vi "e.gate Decode Summary File.vi"(8 "error in (no error)":errorcluster, 11 "e.gate Configuration In":T1) -> (0 "error out":errorcluster, 3 "e.gate Configuration Out":T1)   [LabVIEW 2016]
doc: "This VI reads all, for decoding relevant, data from #summary.sta ini file to the configuration cluster."
uses:
  e.gate Configuration.ctl
  e.gate Channel Data.ctl
  e.gate Data Type.ctl
  e.gate Protocol Type.ctl
  e.gate Module  Data.ctl
  e.gateHSP_DLLhandle.ctl
  <vilib>/Utility/config.llb/Read Key (String).vi
  <vilib>/Utility/config.llb/NI_LVConfig.lvlib
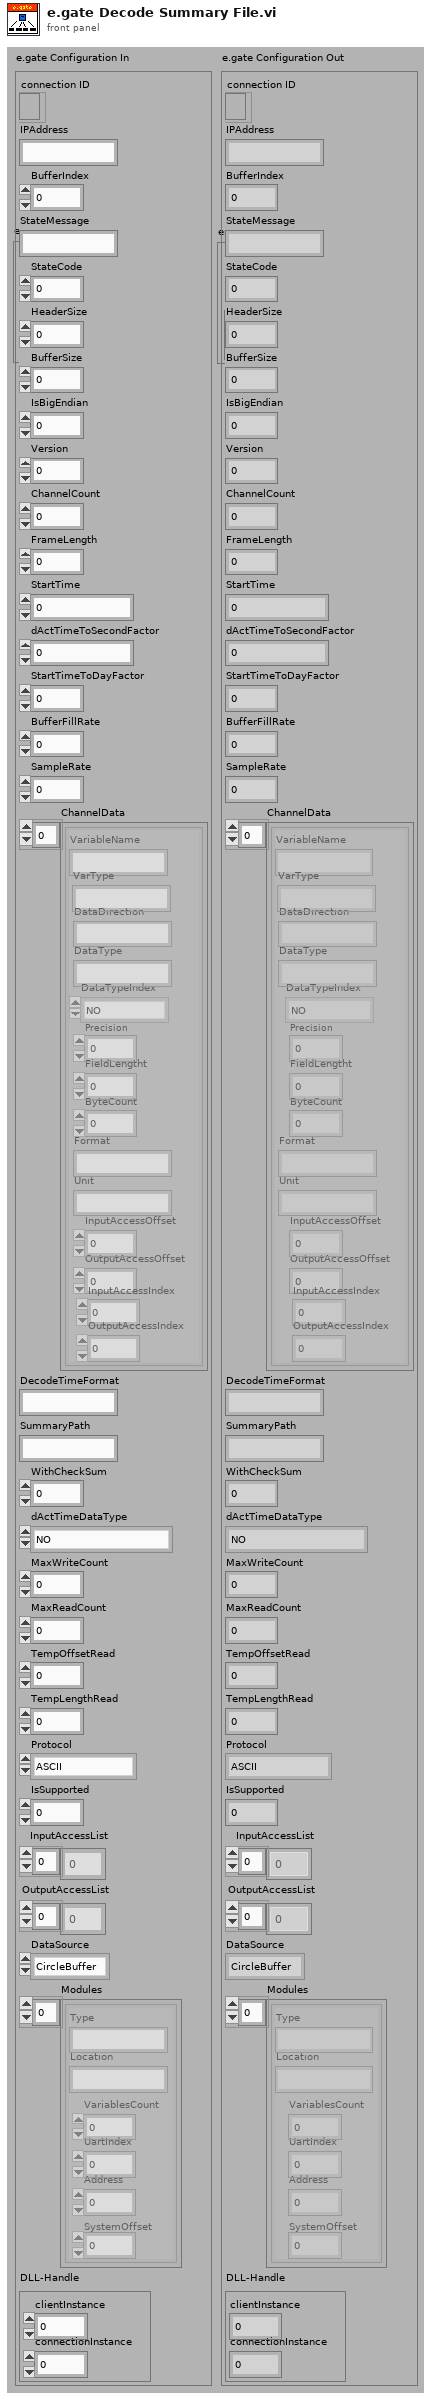
[diagram p1: front panel]
types:
  T1 = typedef "e.gate Configuration.ctl" = cluster{"connection ID":refnum<k5>, "IPAddress":string, "BufferIndex":i32, "StateMessage":string, "StateCode":i8, "HeaderSize":i32, "BufferSize":i32, "IsBigEndian":i32, "Version":i32, "ChannelCount":i32, "FrameLength":i32, "StartTime":dbl, "dActTimeToSecondFactor":dbl, "StartTimeToDayFactor":dbl, "BufferFillRate":dbl, "SampleRate":dbl, "ChannelData":T2[], "DecodeTimeFormat":string, "SummaryPath":string, "WithCheckSum":i32, "dActTimeDataType":T3, "MaxWriteCount":i32, "MaxReadCount":i32, "TempOffsetRead":i32, "TempLengthRead":i32, "Protocol":T4, "IsSupported":i32, "InputAccessList":i32[], "OutputAccessList":i32[], "DataSource":enum16{"CircleBuffer", "test.con Logger", "test.con Archive"}, "Modules":T5[], "DLL-Handle":T6}
  T2 = typedef "e.gate Channel Data.ctl" = cluster{"VariableName":string, "DataDirection":string, "DataType":string, "DataTypeIndex":T3, "Precision":i16, "FieldLengtht":i16, "ByteCount":i32, "Format":string, "Unit":string, "InputAccessOffset":i32, "OutputAccessOffset":i16, "InputAccessIndex":i16, "OutputAccessIndex":i16, "VarType":string}
  T3 = typedef "e.gate Data Type.ctl" = enum16{"NO", "BOOL", "SINT8", "USINT8", "SINT16", "USINT16", "SINT32", "USINT32", "FLOAT", "SET8", "SET16", "SET32", "DOUBLE", "SINT64", "USINT64", "SET64"}
  T4 = typedef "e.gate Protocol Type.ctl" = enum16{"ASCII", "HighspeedPort Online", "HighspeedPort Buffer", "eGateHighspeedPortDLL "}
  T5 = typedef "e.gate Module  Data.ctl" = cluster{"Type":string, "Location":string, "VariablesCount":i16, "UartIndex":i16, "Address":i16, "SystemOffset":i16}
  T6 = typedef "e.gateHSP_DLLhandle.ctl" = cluster{"clientInstance":i32, "connectionInstance":i32}
  T7 = typedef "NI_LVConfig.lvlib/Config Data RefNum.ctl" = refnum<k1>
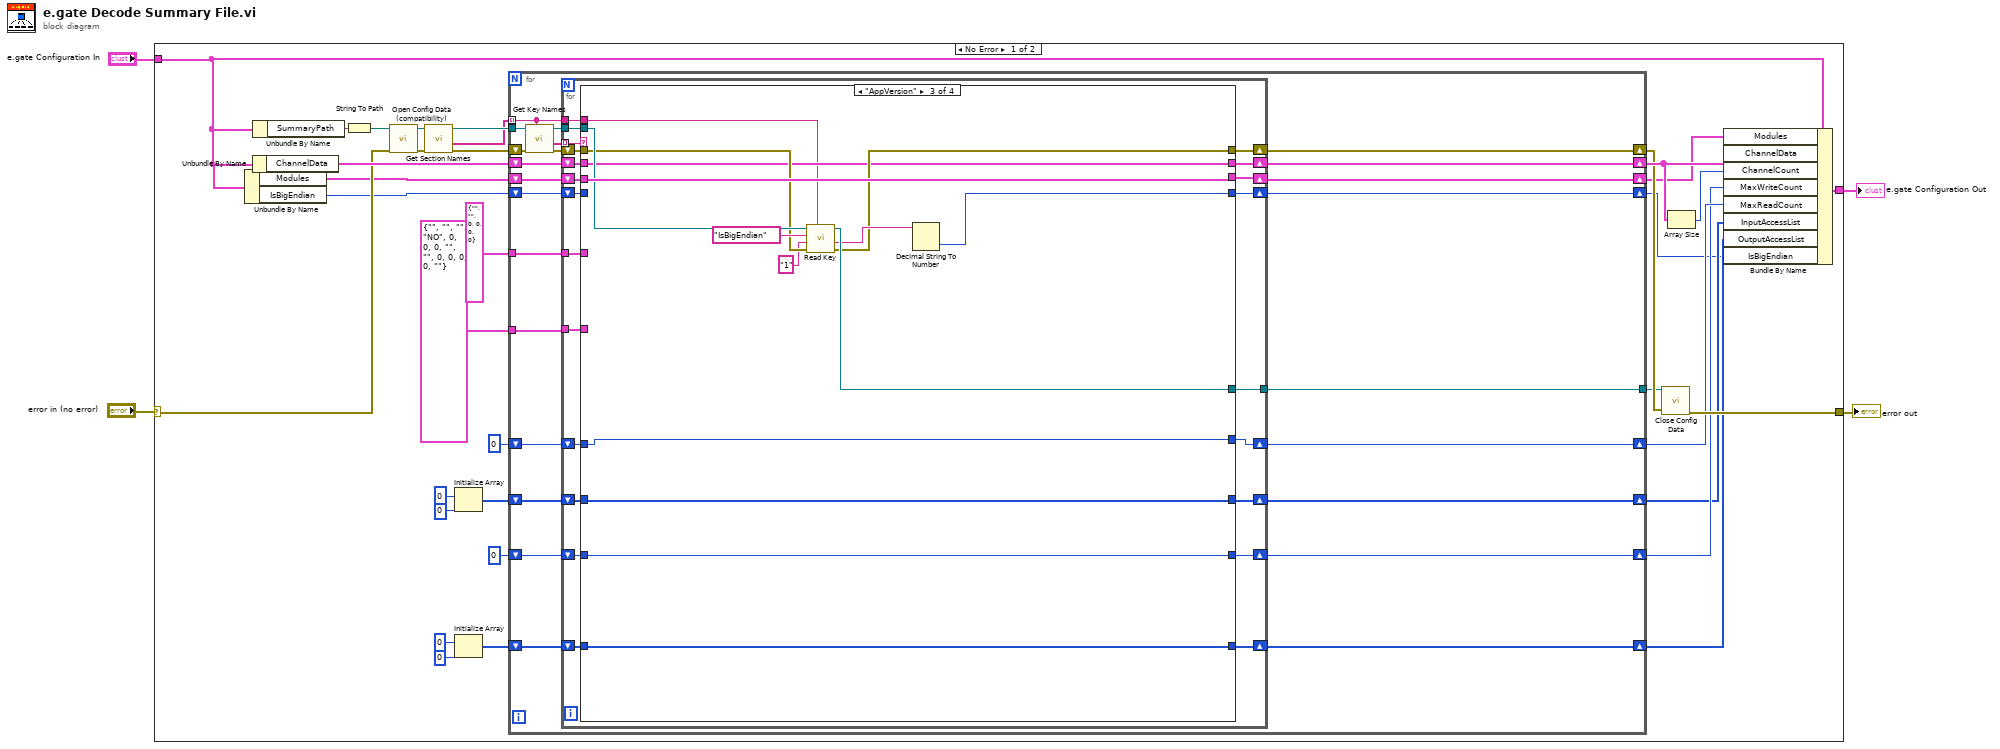
[diagram p0: block diagram]
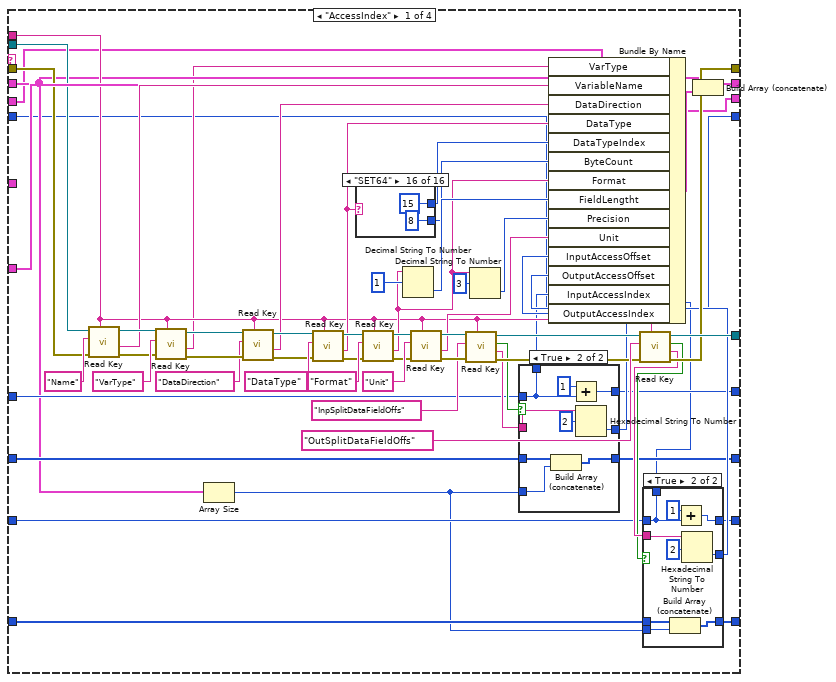
[diagram p2: hidden frame]
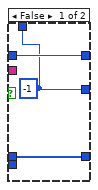
[diagram p3: hidden frame]
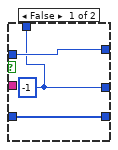
[diagram p4: hidden frame]
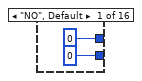
[diagram p5: hidden frame]
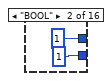
[diagram p6: hidden frame]
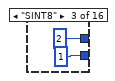
[diagram p7: hidden frame]
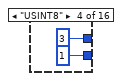
[diagram p8: hidden frame]
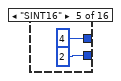
[diagram p9: hidden frame]
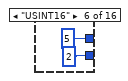
[diagram p10: hidden frame]
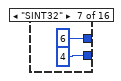
[diagram p11: hidden frame]
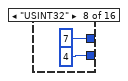
[diagram p12: hidden frame]
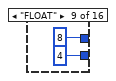
[diagram p13: hidden frame]
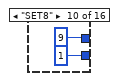
[diagram p14: hidden frame]
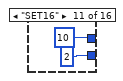
[diagram p15: hidden frame]
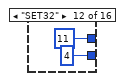
[diagram p16: hidden frame]
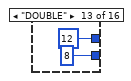
[diagram p17: hidden frame]
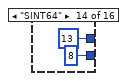
[diagram p18: hidden frame]
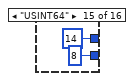
[diagram p19: hidden frame]
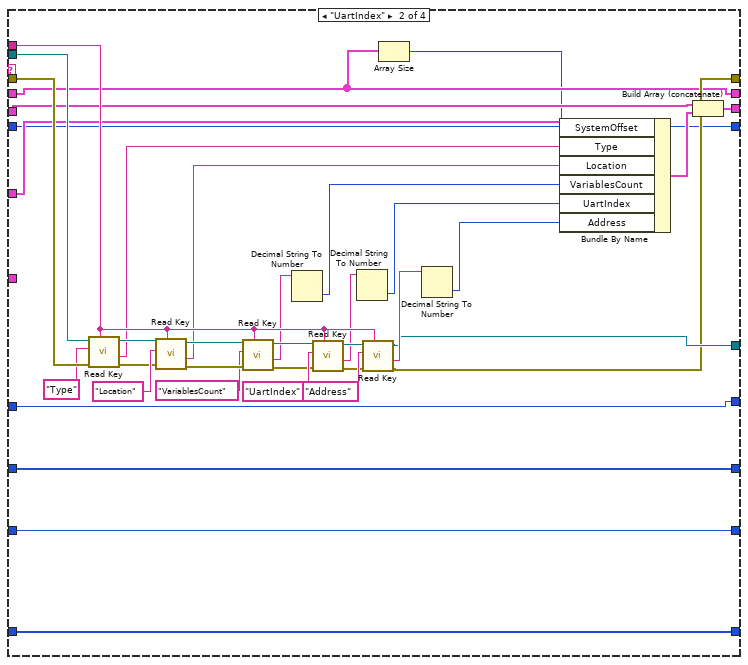
[diagram p20: hidden frame]
diagram:
  n1 = case shown="No Error" "error in (no error)" {
    selector: "error in (no error)" -> [w27 w264]
    tunnel: "e.gate Configuration In" -> [w11 w265]
    tunnel: [w14 w265] -> w2
    tunnel: [w30 w264] -> w1
    frame No Error {
      n2 = Unbundle By Name(w11) -> ("Modules"=w9:T5[], "IsBigEndian"=w6:i32)
      n3 = Unbundle By Name(w11) -> ("ChannelData"=w31:T2[])
      n4 = Unbundle By Name(w11) -> ("SummaryPath"=w36:string)
      n5 = String To Path(string=w36) -> (path=w28:path)
      n6 = call <vilib>:"Open Config Data (compatibility).vi"("error in (no error)"=w27, "configuration file path"=w28) -> ("error out"=w37:errorcluster, "refnum"=w38:T7)  [unwired: 7 in, 1 out]
      n7 = call <vilib>:"Get Section Names.vi"("error in (no error)"=w37, "refnum"=w38) -> ("error out"=w34:errorcluster, "section names"=w7:string[], "refnum out"=w35:T7)  [unwired: 7 out]
      n8 = Initialize Array(0 ("Element"), 0 ("Dimensionsgröße")) -> (w18:i32[])
      n9 = Initialize Array(0 ("Element"), 0 ("Dimensionsgröße")) -> (w15:i32[])
      n10 = for {
        tunnel: w7 -> [w55] mode=indexing
        tunnel: w35 -> [w62]
        shift-right: [w56] -> w33
        shift-left: w31 -> [w57]
        tunnel: T2 {"VariableName"="", "DataDirection"="", "DataType"="", "DataTypeIndex"=enum."NO", "Precision"=0, "FieldLengtht"=0, "ByteCount"=0, "Format"="", "Unit"="", "InputAccessOffset"=0, "OutputAccessOffset"=0, "InputAccessIndex"=0, "OutputAccessIndex"=0, "VarType"=""} ("Cluster aus Klassenprivatdaten") -> [w54]
        shift-right: [w53] -> w26
        shift-left: w34 -> [w61]
        tunnel: [w52] -> w25
        shift-right: [w51] -> w21
        shift-left: 0 -> [w50]
        shift-right: [w49] -> w22
        shift-left: 0 -> [w48]
        shift-right: [w45] -> w13
        shift-left: w18 -> [w47]
        shift-right: [w44] -> w12
        shift-left: w15 -> [w46]
        tunnel: T5 {"Type"="", "Location"="", "VariablesCount"=0, "UartIndex"=0, "Address"=0, "SystemOffset"=0} ("Mudules") -> [w43]
        shift-right: [w41] -> w8
        shift-left: w9 -> [w42]
        shift-right: [w39] -> w5
        shift-left: w6 -> [w40]
        n11 = call <vilib>:"Get Key Names.vi"("section"=w55, "error in (no error)"=w61, "refnum"=w62) -> ("error out"=w59:errorcluster, "key names"=w60:string[], "refnum out"=w58:T7)  [unwired: 6 out]
        n12 = for {
          tunnel: w60 -> [w78] mode=indexing
          tunnel: w55 -> [w84]
          tunnel: w58 -> [w82]
          tunnel: w54 -> [w79]
          shift-right: [w80] -> w56
          shift-left: w57 -> [w81]
          shift-right: [w77] -> w53
          shift-left: w59 -> [w83]
          tunnel: [w76] -> w52
          shift-right: [w75] -> w51
          shift-left: w50 -> [w74]
          shift-right: [w73] -> w49
          shift-left: w48 -> [w72]
          shift-right: [w69] -> w45
          shift-left: w47 -> [w71]
          shift-right: [w68] -> w44
          shift-left: w46 -> [w70]
          tunnel: w43 -> [w67]
          shift-right: [w65] -> w41
          shift-left: w42 -> [w66]
          shift-right: [w63] -> w39
          shift-left: w40 -> [w64]
          n13 = case shown="\"AppVersion\"" w78 {
            tunnel: w84 -> [w103 w225 w241 _]
            tunnel: w83 -> [w105 w227 w244 w262]
            tunnel: w82 -> [w104 w226 w249 w263]
            tunnel: [w110 w206 w243 w262] -> w77
            tunnel: [w111 w207 w247 w263] -> w76
            tunnel: w81 -> [w91 w205 w242 w261]
            tunnel: [w117 w205 w242 w261] -> w80
            tunnel: w79 -> [w115 _ _ _]
            tunnel: [w99 w218 w254 w260] -> w75
            tunnel: w74 -> [w92 w218 w254 w260]
            tunnel: [w98 w220 w253 w259] -> w73
            tunnel: w72 -> [w97 w220 w253 w259]
            tunnel: w71 -> [w96 w219 w252 w258]
            tunnel: w70 -> [w94 w217 w251 w257]
            tunnel: [w95 w219 w252 w258] -> w69
            tunnel: [w93 w217 w251 w257] -> w68
            tunnel: w67 -> [_ w224 _ _]
            tunnel: w66 -> [w87 w223 w250 w256]
            tunnel: [w87 w222 w250 w256] -> w65
            tunnel: w64 -> [w85 w203 _ w255]
            tunnel: [w85 w203 w245 w255] -> w63
            frame "AccessIndex" {
              n14 = call-poly <vilib>:"Read Key.vi"("section"=w103, "error in (no error)"=w105, "key"="Name" ("section"), "refnum"=w104) -> ("error out"=w144:errorcluster, "value"=w127:string, "refnum out"=w143:T7)  [unwired: 2 in, 3 out]
              n15 = call-poly <vilib>:"Read Key.vi"("section"=w103, "error in (no error)"=w144, "key"="VarType" ("section"), "refnum"=w143) -> ("error out"=w141:errorcluster, "value"=w86:string, "refnum out"=w142:T7)  [unwired: 2 in, 3 out]
              n16 = Array Size(array=w91) -> (size(s)=w90:i32)
              n17 = call-poly <vilib>:"Read Key.vi"("section"=w103, "error in (no error)"=w141, "key"="DataDirection" ("section"), "refnum"=w142) -> ("error out"=w135:errorcluster, "value"=w126:string, "refnum out"=w131:T7)  [unwired: 2 in, 3 out]
              n18 = call-poly <vilib>:"Read Key.vi"("section"=w103, "error in (no error)"=w135, "key"="DataType", "refnum"=w131) -> ("error out"=w134:errorcluster, "value"=w125:string, "refnum out"=w130:T7)  [unwired: 2 in, 3 out]
              n19 = case shown="\"SET64\"" w125 {
                tunnel: [i16 0 ("Precision") i16 1 ("Precision") 1 1 ("Precision") 2 ("Precision") 2 ("Precision") 4 ("Precision") 4 ("Precision") 4 ("Precision") 1 ("Precision") 2 ("Precision") 4 ("Precision") i16 8 ("Precision") 8 ("Precision") 8 ("Precision") 8 ("Precision")] -> w116
                tunnel: [i16 0 ("Precision") i16 1 ("Precision") i16 2 ("Precision") i16 3 ("Precision") i16 4 ("Precision") i16 5 ("Precision") i16 6 ("Precision") i16 7 ("Precision") i16 8 ("Precision") i16 9 ("Precision") i16 10 ("Precision") i16 11 ("Precision") i16 12 ("Precision") i16 13 ("Precision") i16 14 ("Precision") i16 15 ("Precision")] -> w124
                frame "NO", Default {
                }
                frame "BOOL" {
                }
                frame "SINT8" {
                }
                frame "USINT8" {
                }
                frame "SINT16" {
                }
                frame "USINT16" {
                }
                frame "SINT32" {
                }
                frame "USINT32" {
                }
                frame "FLOAT" {
                }
                frame "SET8" {
                }
                frame "SET16" {
                }
                frame "SET32" {
                }
                frame "DOUBLE" {
                }
                frame "SINT64" {
                }
                frame "USINT64" {
                }
                frame "SET64" {
                }
              }
              n20 = call-poly <vilib>:"Read Key.vi"("section"=w103, "error in (no error)"=w134, "key"="Format", "refnum"=w130) -> ("error out"=w133:errorcluster, "value"=w119:string, "refnum out"=w129:T7)  [unwired: 2 in, 3 out]
              n21 = Decimal String To Number(string=w119, offset=1 ("Offset")) -> (number=w122:i32)  [unwired: 2 out]
              n22 = call-poly <vilib>:"Read Key.vi"("section"=w103, "error in (no error)"=w133, "key"="Unit", "refnum"=w129) -> ("error out"=w132:errorcluster, "value"=w118:string, "refnum out"=w128:T7)  [unwired: 2 in, 3 out]
              n23 = call-poly <vilib>:"Read Key.vi"("section"=w103, "error in (no error)"=w132, "key"="InpSplitDataFieldOffs", "refnum"=w128) -> ("error out"=w112:errorcluster, "value"=w109:string, "found?"=w102:bool, "refnum out"=w113:T7)  [unwired: 2 in, 2 out]
              n24 = Decimal String To Number(string=w119, offset=3 ("Offset")) -> (number=w121:i32)  [unwired: 2 out]
              n25 = case shown="True" w102 {
                tunnel: w109 -> [_ w170]
                tunnel: [w159 w169] -> w107
                tunnel: [w161 w167] -> w98
                tunnel: w97 -> [w161 w162]
                tunnel: w96 -> [w160 w165]
                tunnel: [w160 w164] -> w95
                tunnel: w90 -> [_ w163]
                tunnel: [w159 w162] -> w88
                frame False {
                  w159 = -1
                }
                frame True {
                  n26 = Build Array (concatenate)(w165, w163) -> (w164:i32[])
                  n27 = Add(x=1, y=w162) -> (x+y=w167:i32)
                  n28 = Hexadecimal String To Number(string=w170, offset=2) -> (number=w169:u32)  [unwired: 2 out]
                }
              }
              n29 = call-poly <vilib>:"Read Key.vi"("section"=w103, "error in (no error)"=w112, "key"="OutSplitDataFieldOffs", "refnum"=w113) -> ("error out"=w110:errorcluster, "value"=w108:string, "found?"=w101:bool, "refnum out"=w111:T7)  [unwired: 2 in, 2 out]
              n30 = case shown="True" w101 {
                tunnel: w108 -> [_ w158]
                tunnel: [w147 w156] -> w106
                tunnel: [w149 w155] -> w99
                tunnel: w92 -> [w149 w150]
                tunnel: w94 -> [w148 w152]
                tunnel: [w148 w153] -> w93
                tunnel: w90 -> [_ w151]
                tunnel: [w147 w150] -> w89
                frame False {
                  w147 = -1
                }
                frame True {
                  n31 = Build Array (concatenate)(w152, w151) -> (w153:i32[])
                  n32 = Add(x=1, y=w150) -> (x+y=w155:i32)
                  n33 = Hexadecimal String To Number(string=w158, offset=2) -> (number=w156:u32)  [unwired: 2 out]
                }
              }
              n34 = Bundle By Name(cluster=w115, "VarType"=w86, "VariableName"=w127, "DataDirection"=w126, "DataType"=w125, "DataTypeIndex"=w124, "ByteCount"=w116, "Format"=w119, "FieldLengtht"=w122, "Precision"=w121, "Unit"=w118, "InputAccessOffset"=w107, "OutputAccessOffset"=w106, "InputAccessIndex"=w88, "OutputAccessIndex"=w89) -> (w100:T2)
              n35 = Build Array (concatenate)(w91, w100) -> (w117:T2[])
            }
            frame "UartIndex" {
              n36 = call-poly <vilib>:"Read Key.vi"("section"=w225, "error in (no error)"=w227, "key"="Type", "refnum"=w226) -> ("error out"=w238:errorcluster, "value"=w215:string, "refnum out"=w237:T7)  [unwired: 2 in, 3 out]
              n37 = call-poly <vilib>:"Read Key.vi"("section"=w225, "error in (no error)"=w238, "key"="Location" ("section"), "refnum"=w237) -> ("error out"=w235:errorcluster, "value"=w214:string, "refnum out"=w236:T7)  [unwired: 2 in, 3 out]
              n38 = call-poly <vilib>:"Read Key.vi"("section"=w225, "error in (no error)"=w235, "key"="VariablesCount" ("section"), "refnum"=w236) -> ("error out"=w231:errorcluster, "value"=w213:string, "refnum out"=w229:T7)  [unwired: 2 in, 3 out]
              n39 = Decimal String To Number(string=w213) -> (number=w212:i32)  [unwired: 1 in, 2 out]
              n40 = call-poly <vilib>:"Read Key.vi"("section"=w225, "error in (no error)"=w231, "key"="UartIndex", "refnum"=w229) -> ("error out"=w230:errorcluster, "value"=w211:string, "refnum out"=w228:T7)  [unwired: 2 in, 3 out]
              n41 = Decimal String To Number(string=w211) -> (number=w210:i32)  [unwired: 1 in, 2 out]
              n42 = call-poly <vilib>:"Read Key.vi"("section"=w225, "error in (no error)"=w230, "key"="Address", "refnum"=w228) -> ("error out"=w206:errorcluster, "value"=w209:string, "refnum out"=w207:T7)  [unwired: 2 in, 3 out]
              n43 = Array Size(array=w205) -> (size(s)=w204:i32)
              n44 = Decimal String To Number(string=w209) -> (number=w208:i32)  [unwired: 1 in, 2 out]
              n45 = Bundle By Name(cluster=w224, "SystemOffset"=w204, "Type"=w215, "Location"=w214, "VariablesCount"=w212, "UartIndex"=w210, "Address"=w208) -> (w221:T5)
              n46 = Build Array (concatenate)(w223, w221) -> (w222:T5[])
            }
            frame "AppVersion" {
              n47 = call-poly <vilib>:"Read Key.vi"("section"=w241, "error in (no error)"=w244, "default value"="1", "key"="IsBigEndian", "refnum"=w249) -> ("error out"=w243:errorcluster, "value"=w246:string, "refnum out"=w247:T7)  [unwired: 1 in, 3 out]
              n48 = Decimal String To Number(string=w246) -> (number=w245:i32)  [unwired: 1 in, 2 out]
            }
            frame "default", Default {
            }
          }
        }
      }
      n49 = call <vilib>:"Close Config Data.vi"("error in (no error)"=w26, "refnum"=w25) -> ("error out"=w30:errorcluster)  [unwired: 1 in, 8 out]
      n50 = Array Size(array=w33) -> (size(s)=w32:i32)
      n51 = Bundle By Name(cluster=w11, "Modules"=w8, "ChannelData"=w33, "ChannelCount"=w32, "MaxWriteCount"=w21, "MaxReadCount"=w22, "InputAccessList"=w13, "OutputAccessList"=w12, "IsBigEndian"=w5) -> (w14:T1)
    }
    frame Error {
    }
  }
  "e.gate Configuration Out" <- w2
  "error out" <- w1
